vi "Asynchronous - Acyclic Channels - Send.vi"(4 "Raw Values Array":u32[](array[numeric]), 5 "Channel Data []":T5[](array[typedef])=[{"Labels Settings"=[{"Name"="", "xmlName"="", "Label"=0, "transferPeriod"=0, "SDI_Enabled"=FALSE, "SDI"=0, "Word"={"Param Setting"={"Start Bit"=[], "Num Bits"=[], "Signed?"=[], "ScaleFac"=[], "ScaleOffset"=[], "Block Data Refs"=[], "Encoding"=[], "Values Array"=[], "Item Refs"=[]}}, "TransferType"=enum."ScheduledLabel", "has timestamp?"=FALSE, "Label Disable/Trigger Channel Reference"=0, "Message Handle"=0, "Initialized?"=FALSE, "Word Initial Raw Value"=0, "Label Timestamp Channel Data Reference"=0}], "channel handle"=0, "channel #"=0}] {"Labels Settings"."Label Timestamp Channel Data Reference" format="%.0x"; "Labels Settings"."Label Disable/Trigger Channel Reference" format="%.0x"; "Labels Settings"."Word"."Param Setting"."Item Refs" format="%.0x"; "Labels Settings"."Word"."Param Setting"."Num Bits" min=1 max=32; "Labels Settings"."Word"."Param Setting"."Start Bit" min=8 max=31; "Labels Settings"."Label" format="%.0o"}, 6 "Raw Values Index Array":i32[](array[numeric]), 7 "Tx Map - Trigger Channels":T4[](array[typedef]) {"Channel Data Reference" format="%.0x"}, 8 "Error (in)":errorcluster, 11 "Changes?":bool[](array[boolean])) -> (0 "Error (out)":errorcluster)   [LabVIEW 2020, in "Ballard Arinc-429 Engine.lvlib"]
uses:
  Ballard Arinc-429 Engine.lvlib
  Shared/Controls and Global/RT HW Channel.ctl
  Shared/Controls and Global/RT Label Settings.ctl
  Shared/Controls and Global/Label.ctl
  Shared/Controls and Global/transferPeriod.ctl
  Shared/Controls and Global/RT Word Settings.ctl
  Shared/Controls and Global/RT Param Setting.ctl
  Shared/Controls and Global/Start Bit.ctl
  Shared/Controls and Global/Number of Bits.ctl
  <vilib>/NI VeriStand/Custom Device API/Block Data Reference.ctl
  <vilib>/NI VeriStand/Custom Device API/Data Reference.ctl
  <vilib>/NI VeriStand/Custom Device API/Custom Device Item Ref.ctl
  Shared/Controls and Global/TransferType.ctl
  RT Controls/RT Tx Association Trigger Channels.ctl
  RT Controls/RT Tx Default Raw Value.ctl
  RT Controls/RT Tx Default Raw Value_Association.ctl
  <instrlib>/BTI429Lib/Private/Tx/Data/Transmit Message Dynamic.vi
  <instrlib>/BTI429Lib/BTI429LV.lvlib
  Shared/Ballard Arinc-429 Shared.lvlib
  <vilib>/NI VeriStand/Custom Device API/Custom Device API.lvlib
panel:
  in  "Acyclic Labels - Raw Values":T1
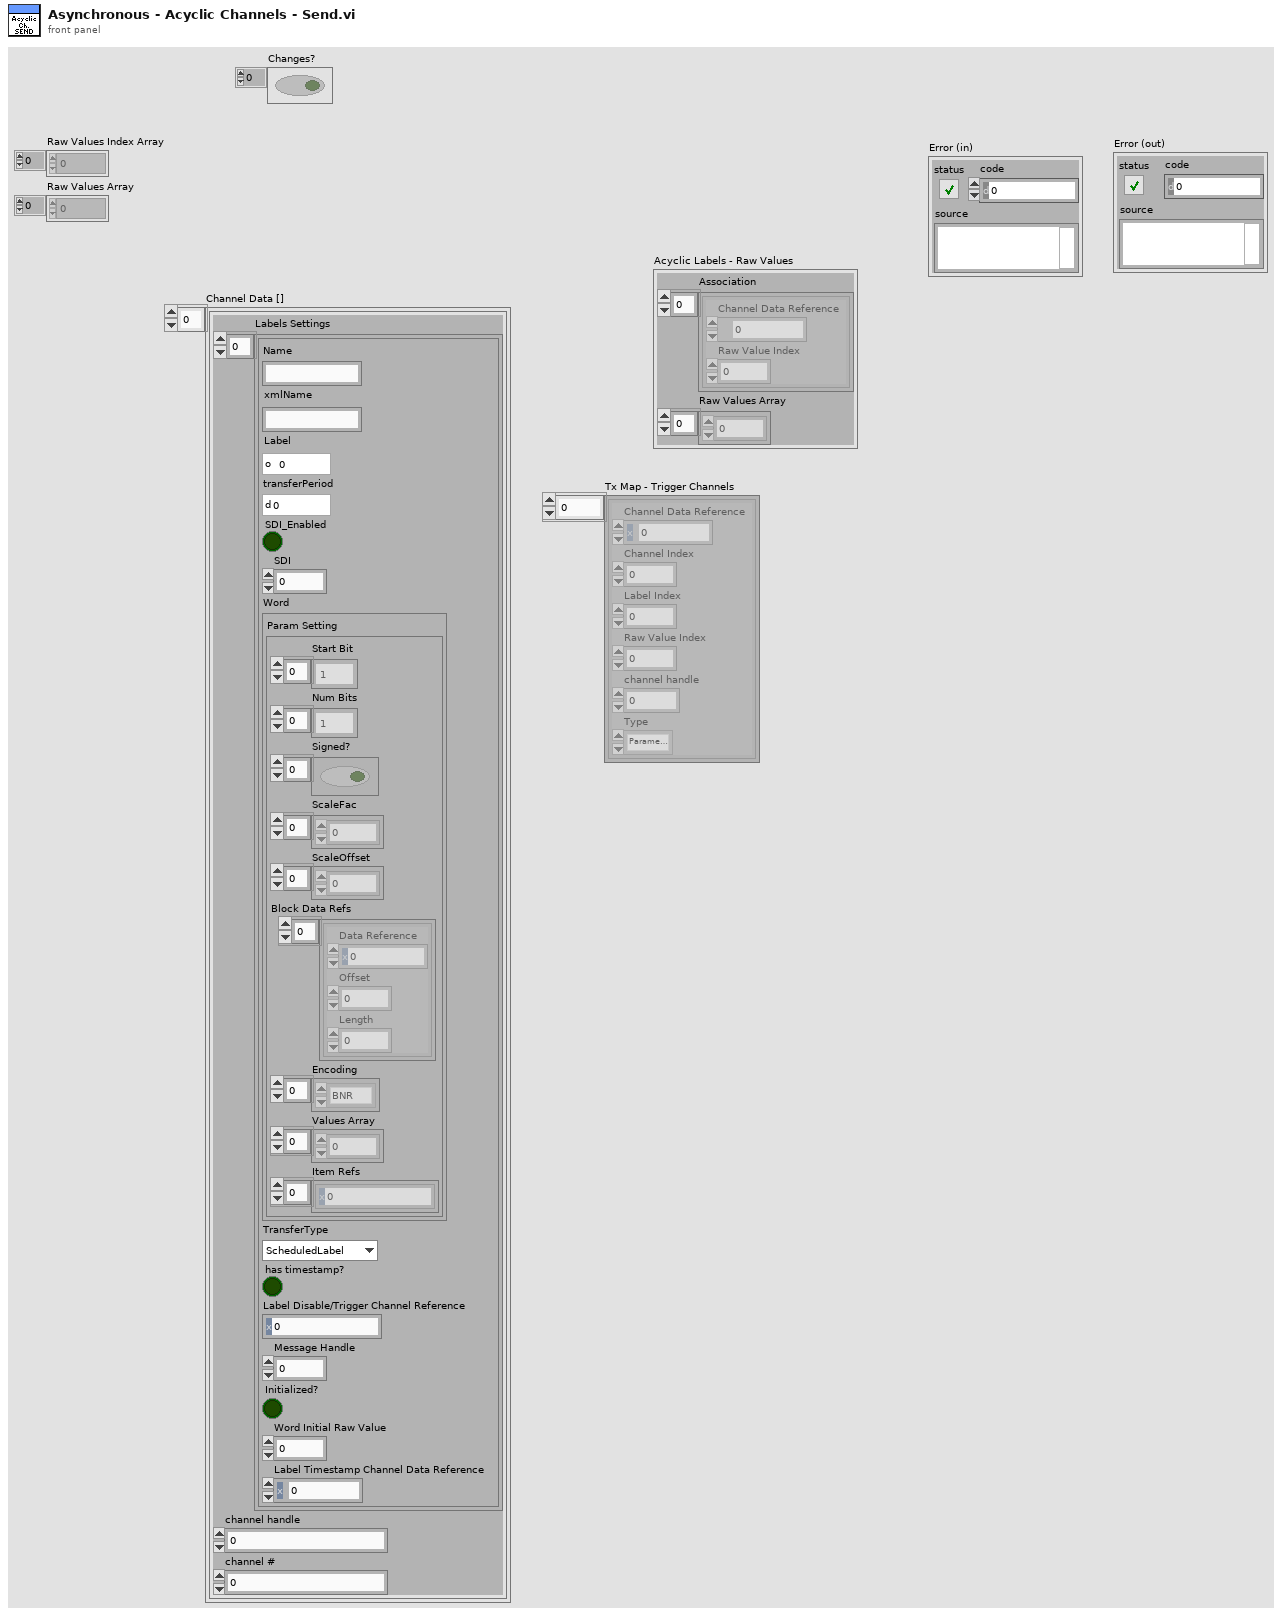
[diagram p1: front panel]
types:
  T1 = typedef "Ballard Arinc-429 Engine.lvlib/RT Tx Default Raw Value.ctl" = cluster{"Association":T2[], "Raw Values Array":u32[]}
  T2 = typedef "Ballard Arinc-429 Engine.lvlib/RT Tx Default Raw Value_Association.ctl" = cluster{"Channel Data Reference":T3, "Raw Value Index":i32}
  T3 = typedef "Custom Device API.lvlib/Data Reference.ctl" = i32
  T4 = typedef "Ballard Arinc-429 Engine.lvlib/RT Tx Association Trigger Channels.ctl" = cluster{"Channel Data Reference":T3, "Channel Index":i32, "Label Index":i32, "Raw Value Index":i32, "channel handle":u64, "Type":enum16{"Parameter Channel", "Disable/Trigger Channel"}}
  T5 = typedef "Ballard Arinc-429 Shared.lvlib/RT HW Channel.ctl" = cluster{"Labels Settings":T6[], "channel handle":u64, "channel #":u16}
  T6 = typedef "Ballard Arinc-429 Shared.lvlib/RT Label Settings.ctl" = cluster{"Name":string, "xmlName":string, "Label":T7, "transferPeriod":T8, "SDI_Enabled":bool, "SDI":u8, "Word":T9, "TransferType":T15, "has timestamp?":bool, "Label Disable/Trigger Channel Reference":T14, "Message Handle":u64, "Initialized?":bool, "Word Initial Raw Value":u32, "Label Timestamp Channel Data Reference":T3}
  T7 = typedef "Ballard Arinc-429 Shared.lvlib/Label.ctl" = u8
  T8 = typedef "Ballard Arinc-429 Shared.lvlib/transferPeriod.ctl" = u32
  T9 = typedef "Ballard Arinc-429 Shared.lvlib/RT Word Settings.ctl" = cluster{"Param Setting":T10}
  T10 = typedef "Ballard Arinc-429 Shared.lvlib/RT Param Setting.ctl" = cluster{"Start Bit":T11[], "Num Bits":T12[], "Signed?":bool[], "ScaleFac":dbl[], "ScaleOffset":dbl[], "Block Data Refs":T13[], "Encoding":enum16{"BNR", "BCD", "Discrete"}[], "Values Array":dbl[], "Item Refs":T14[]}
  T11 = typedef "Ballard Arinc-429 Shared.lvlib/Start Bit.ctl" = i32
  T12 = typedef "Ballard Arinc-429 Shared.lvlib/Number of Bits.ctl" = i32
  T13 = typedef "Custom Device API.lvlib/Block Data Reference.ctl" = cluster{"Data Reference":T3, "Offset":u64, "Length":u64}
  T14 = typedef "Custom Device API.lvlib/Custom Device Item Ref.ctl" = u64
  T15 = typedef "Ballard Arinc-429 Shared.lvlib/TransferType.ctl" = enum16{"ScheduledLabel", "Acyclic", "Block", "Strobe"}
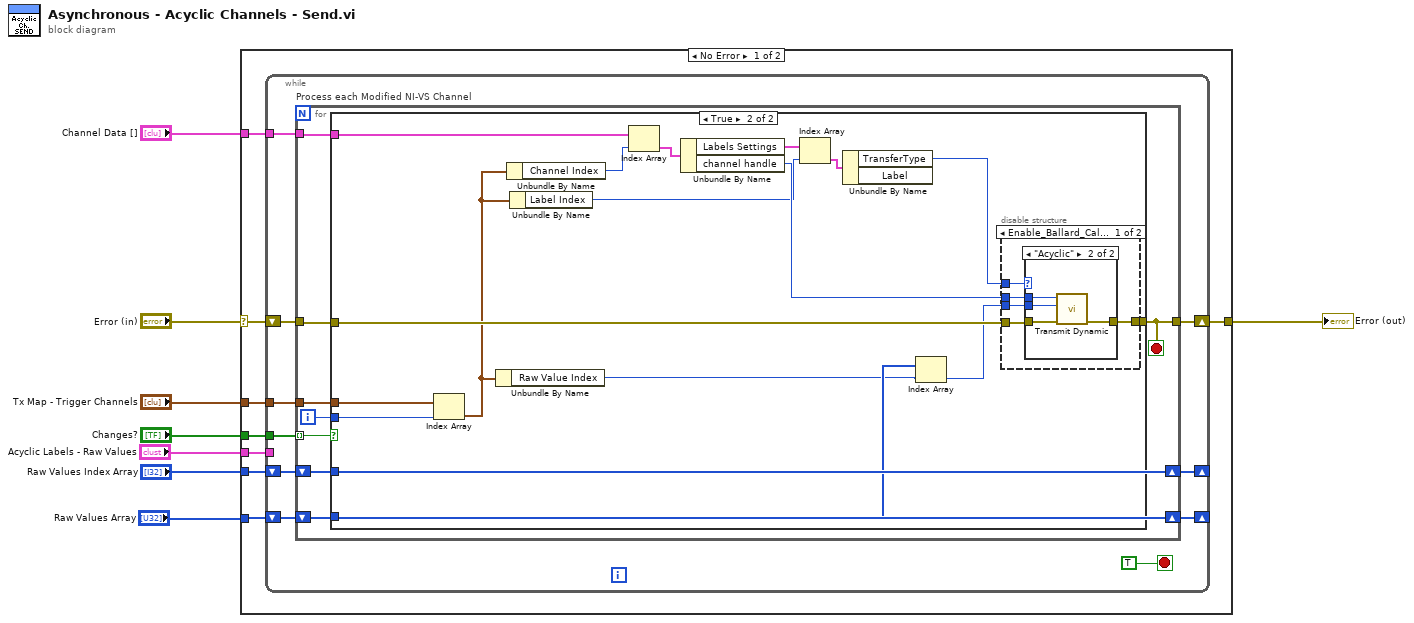
[diagram p0: block diagram]
diagram:
  n1 = case shown="No Error" "Error (in)" {
    selector: "Error (in)" -> [w12 w63]
    tunnel: "Channel Data []" -> [w16 _]
    tunnel: "Changes?" -> [w15 _]
    tunnel: [w14 w63] -> w6
    tunnel: "Tx Map - Trigger Channels" -> [w13 _]
    tunnel: "Acyclic Labels - Raw Values" -> [w11 _]
    tunnel: "Raw Values Index Array" -> [w10 _]
    tunnel: "Raw Values Array" -> [w9 _]
    frame No Error {
      n2 = while {
        tunnel: w16 -> [w26]
        tunnel: w15 -> [w25]
        tunnel: w13 -> [w22]
        shift-right: [w23] -> w14
        shift-left: w12 -> [w24]
        shift-right: [w20] -> _
        shift-left: w9 -> [w17]
        shift-right: [w19] -> _
        shift-left: w10 -> [w18]
        tunnel: w11 -> [_]
        stop <- TRUE stop-if-true
        n3 = for "Process each Modified NI-VS Channel" {
          tunnel: w26 -> [w33]
          tunnel: w25 -> [w27] mode=indexing
          tunnel: w24 -> [w34]
          tunnel: [w31] -> w23
          tunnel: w22 -> [w32]
          shift-right: [w29] -> w20
          shift-left: w17 -> [w29]
          shift-right: [w30] -> w19
          shift-left: w18 -> [w30]
          i -> [w28]
          stop <- w31 stop-if-true
          n4 = case shown="True" w27 {
            tunnel: w34 -> [w35 w51]
            tunnel: w33 -> [_ w50]
            tunnel: w32 -> [_ w47]
            tunnel: [w35 w46] -> w31
            tunnel: w30 -> [_ _]
            tunnel: w29 -> [_ w45]
            tunnel: w28 -> [_ w39]
            frame False {
            }
            frame True {
              n5 = Index Array(array=w47, index=w39) -> (element=w38:T4)
              n6 = Unbundle By Name(w38) -> ("Raw Value Index"=w37:i32)
              n7 = Unbundle By Name(w38) -> ("Channel Index"=w41:i32)
              n8 = Unbundle By Name(w38) -> ("Label Index"=w40:i32)
              n9 = Index Array(array=w50, index=w41) -> (element=w44:T5)
              n10 = Unbundle By Name(w44) -> ("Labels Settings"=w49:T6[], "channel handle"=w42:u64)
              n11 = Index Array(array=w49, index=w40) -> (element=w48:T6)
              n12 = Unbundle By Name(w48) -> ("TransferType"=w43:T15)  [unwired: 1 out]
              n13 = Index Array(array=w45, index=w37) -> (element=w36:u32)
              n14 = disable-structure shown="Enable_Ballard_Calls==True, Default" {
                disable-tunnel: w51 -> [w56 w62]
                disable-tunnel: [w55 w62] -> w46
                disable-tunnel: w36 -> [w54 _]
                disable-tunnel: w42 -> [w53 _]
                disable-tunnel: w43 -> [w52 _]
                frame condition #0 (active) {
                  n15 = case shown="\"Acyclic\"" w52 {
                    tunnel: w56 -> [w57 w61]
                    tunnel: [w57 w60] -> w55
                    tunnel: w54 -> [_ w59]
                    tunnel: w53 -> [_ w58]
                    frame "ScheduledLabel", Default {
                    }
                    frame "Acyclic" {
                      n16 = call-poly <instrlib>:"Transmit Dynamic.vi"("error in (no error)"=w61, "message data"=w59, "channel handle in"=w58) -> ("error out"=w60:errorcluster)  [unwired: 7 in, 1 out]
                    }
                  }
                }
                frame condition #1 {
                }
              }
            }
          }
        }
      }
    }
    frame Error {
    }
  }
  "Error (out)" <- w6
